vi "ProcessSerialData.vi"() -> ()   [LabVIEW 2014]
uses:
  Global Data.vi
panel:
  out "Got Packet?":bool
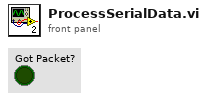
[diagram p1: front panel]
types:
  T1 = typedef "WPI_SerialPortRef.ctl" = cluster{"DevStatus":errorcluster, "Serial Port Name":refnum<visa-resource-name>}
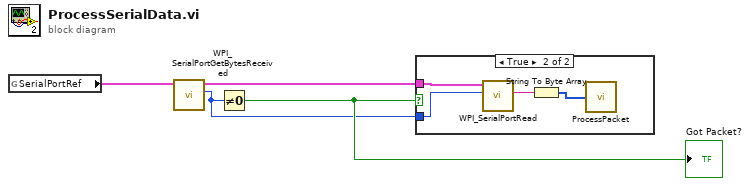
[diagram p0: block diagram]
diagram:
  n1 = global read "Global Data.vi" "SerialPortRef"() -> (w4:T1)
  n2 = call <vilib>:"WPI_SerialPortGetBytesReceived.vi"("SerialPortRef"=w4) -> ("Bytes at Port"=w1:u32, "SerialPortRef"=w2:T1)  [unwired: 8 in, 1 out]
  n3 = Not Equal To 0?(x=w1) -> (x != 0?=w3:bool)
  "Got Packet?" <- w3
  n4 = case shown="True" w3 {
    tunnel: w2 -> [_ w8]
    tunnel: w1 -> [_ w7]
    frame False {
    }
    frame True {
      n5 = call <vilib>:"WPI_SerialPortRead.vi"("Num Bytes to Read"=w7, "SerialPortRef"=w8) -> ("Buffer"=w6:string)  [unwired: 7 in, 2 out]
      n6 = String To Byte Array(string=w6) -> (unsigned byte array=w5:u8[])
      n7 = call "ProcessPacket.vi"("Message"=w5) -> ()  [unwired: 5 in]
    }
  }
